vi "Dichtheitstest durchfuehren.vi"(8 "max. Druckanstieg":sgl, 9 "Wartezeit":sgl, 10 "Aktionen":T1=enum."Unterdruck aufbauen", 11 "Druck FT-IR":sgl) -> (0 "Status":string, 1 "Druckabfall":sgl, 2 "Aktionen":T1=enum."Unterdruck aufbauen", 3 "Verstrichene Zeit":sgl, 4 "Fehler":bool)   [LabVIEW 2020, in "Erweiterte Konfig.lvlib"]
uses:
  Erweiterte Konfig.lvlib
  Aktionen Dichtheitstest.ctl
  Schedule Modul/Aktion FGV Testdaten sammeln.ctl
  FGV PID Aktionen.ctl
  Sprachverwaltung/FGV Aktion Tabelle zerlegen.ctl
  Status Dichtheitstest Aktionen.ctl
  PNS/Aktionen FGV Grenzwerte.ctl
  Stoerungen/Stoerungen Messgeraet/Aktionen Kommunikation Stoerung.ctl
  FT-IR/FT-IR.lvlib
  Stoerungen/Stoerungen.lvlib
  Sprachverwaltung/Sprachverwaltung.lvlib
  Amium PNS/AK Kommunikation/AK Kommunikation.lvlib
  Amium PNS/AK Kommunikation/Amium Kommandos verwalten Aktionen.ctl
  Allgemein/allgemeine Sub-VIs.lvlib
  Schedule Modul/Schedule Modul.lvlib
  PNS/PNS.lvlib
  EPA 1065/Dichtheitstest 1065-345/Dichtheitstest 1065-345.lvlib
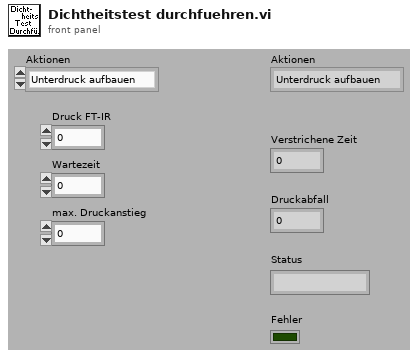
[diagram p1: front panel]
types:
  T1 = typedef "Erweiterte Konfig.lvlib/Aktionen Dichtheitstest.ctl" = enum16{"Initialisieren", "Unterdruck aufbauen", "Prop schließen", "Warten", "Auswertung", "Fertig"}
  T2 = typedef "PNS.lvlib/Aktionen FGV Grenzwerte.ctl" = enum16{"lesen", "Grenzw. schreiben", "Anweisungscode", "IP-Adresse", "laden", "speichern", "Anweisungscode vorgeben"}
  T3 = typedef "Erweiterte Konfig.lvlib/Status Dichtheitstest Aktionen.ctl" = enum16{"lesen", "Zeitstempel", "Daten", "läuft", "Protokolldaten"}
  T4 = typedef "Sprachverwaltung.lvlib/FGV Aktion Tabelle zerlegen.ctl" = enum16{"laden", "vereinzeln", "speichern"}
  T5 = typedef "Erweiterte Konfig.lvlib/FGV PID Aktionen.ctl" = enum16{"Lesen", "Schreiben PID", "Schreiben Sonstige", "Dichtheitstest", "Aktionen Dicht.", "Parameter Sensor"}
  T6 = typedef "Amium PNS.lvlib/AK Kommunikation.lvlib/Amium Kommandos verwalten Aktionen.ctl" = enum16{"lesen", "setzen Ende", "setzen Pos1", "senden", "initalisieren", "prüfen", "Kommandos"}
  T7 = typedef "Schedule Modul.lvlib/Aktion FGV Testdaten sammeln.ctl" = enum16{"lesen", "Dichtheitstest", "CalGasTest", "T90", "Kalibrieren", "init", "Kalender Daten"}
  T8 = typedef "Stoerungen.lvlib/Aktionen Kommunikation Stoerung.ctl" = enum16{"lesen", "init", "FT-IR Komm", "FT-IR Betriebsart", "FT-IR Hintergrund", "cRIO Komm", "PNS Komm", "Dichtheitstest", "Life Bit", "FTIR Komm AK", "PMA Komm", "FID Komm", "PMA Cal", "FID Ch4 Cal", "FID THC Cal", "Cal Timeout", "VFS 1 Komm", "VFS 2 Komm", "VFS 3 Komm", "VFS 4 Komm", "TRE 08 Komm", "CG-Test vorzeitig", "CG-Test Span 1", "CG-Test Span 2", "CG-Test Span 3", "CG-Test Messgas", "CG-Test löschen", "Test", "Amium AK", "AK Recept konfig", "AK Name konfig", "AK EKFG konfig"}
  T9 = typedef "Erweiterte Konfig.lvlib/Sonstige Parameter.ctl" = cluster{"Lüfter langsam":sgl, "Lüfter schnell":sgl, "FT-IR Kühlung Soll":sgl, "FT-IR Kühlung Max":sgl, "Überwachung":T10, "Befüllung aktiv":T11, "Stickstoff Befüllzeit":sgl, "Befüllintervall":sgl, "Kalibrierwert FT-IR":sgl, "Offset Ausgang":sgl, "Offset FT-IR":sgl, "Offset Druck FT-IR":sgl, "Dichtheitstest Zeit":sgl, "Dichtheitstest Abfall":sgl, "Dichtheitstest Umfang":T12, "Offset Umgebung":sgl, "Max Taupunkt":sgl, "Pumpendrehzahl":sgl, "ext. Befüllung":T11, "Ext. Stickstoff Befüllzeit":sgl}
  T10 = typedef "Auswahlfeld.ctl" = u16
  T11 = typedef "LogKonfig.lvlib/Auswahlfeld aktiviert-deaktiviert.ctl" = u16
  T12 = typedef "Erweiterte Konfig.lvlib/Dichtheitstest Umfang.ctl" = u16
  T13 = typedef "Erweiterte Konfig.lvlib/Dichtheitstest Protokoll.ctl" = cluster{"Startzeit":timestamp, "Endzeit":timestamp, "Startdruck":sgl, "Enddruck":sgl, "Dichtheitstest Umfang":T12}
  T14 = typedef "Schedule Modul.lvlib/Ergebnis Dichtheitstest.ctl" = cluster{"Druck FT-IR:":T15, "max. Anstieg:":T15, "Druckanstieg:":T15, "Zeitdauer:":T15, "Verstrichene Zeit:":T15, "Fehler":bool, "Unterdruck nicht erreicht ":bool}
  T15 = typedef "Zahlen-Ausgabefeld.ctl" = sgl
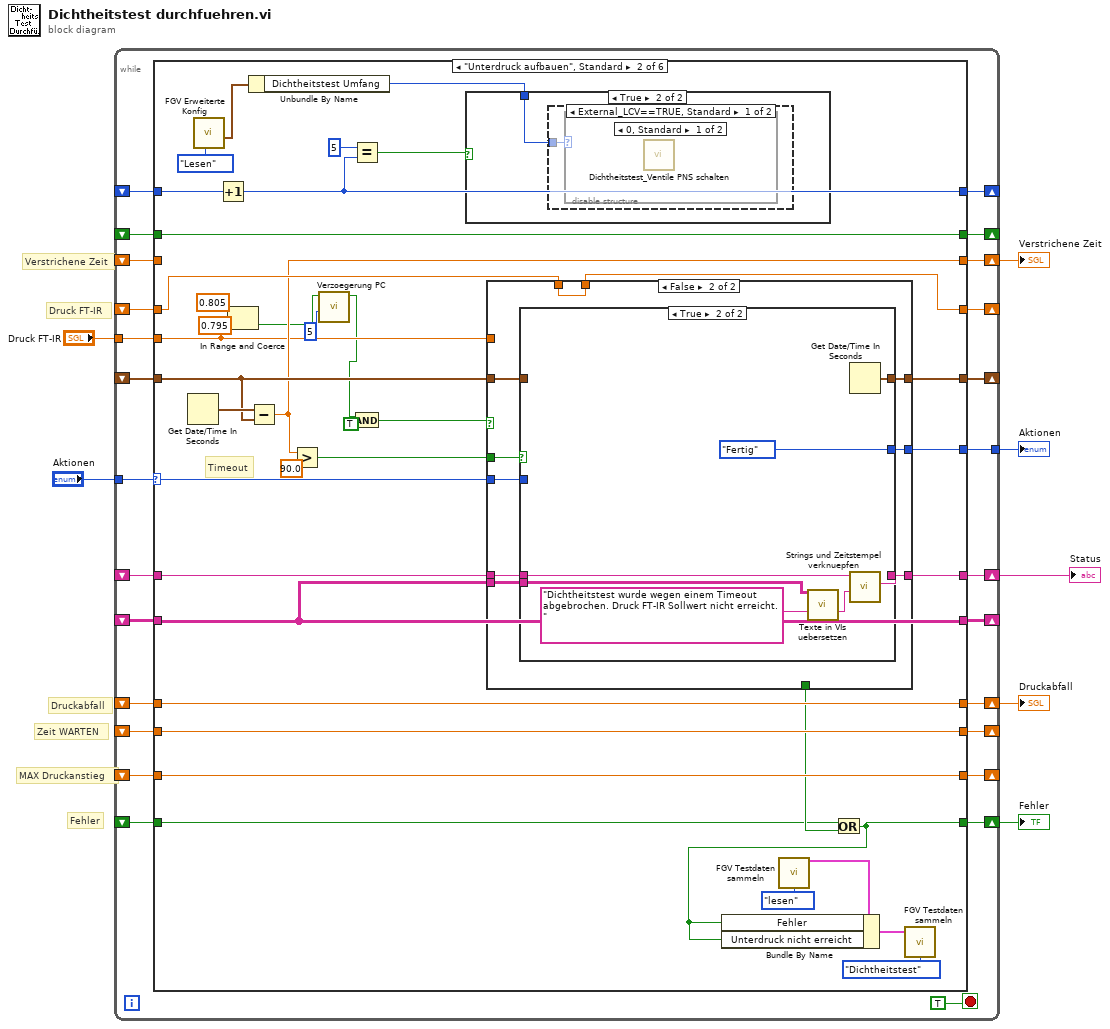
[diagram p0: block diagram]
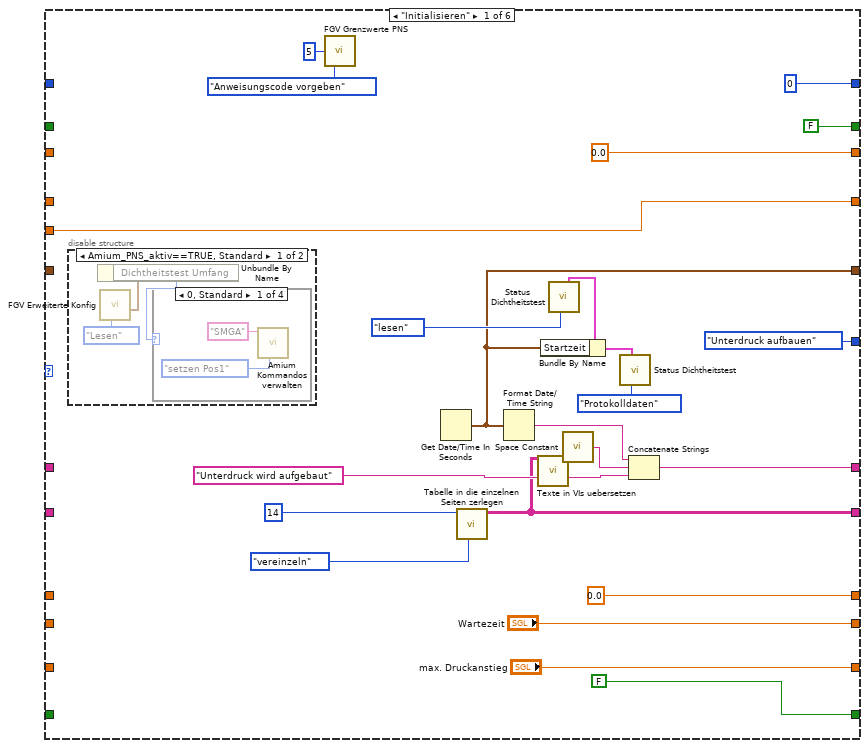
[diagram p2: hidden frame]
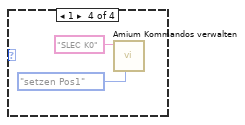
[diagram p5: hidden frame]
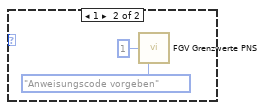
[diagram p8: hidden frame]
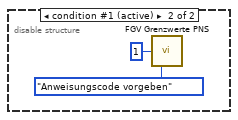
[diagram p9: hidden frame]
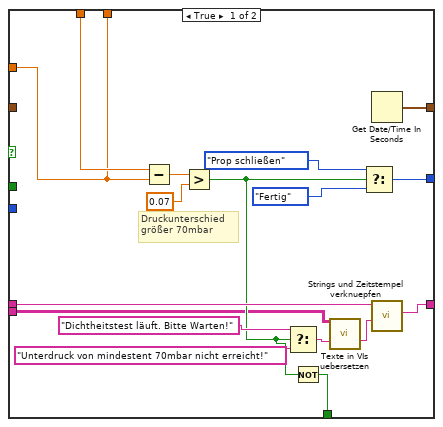
[diagram p10: hidden frame]
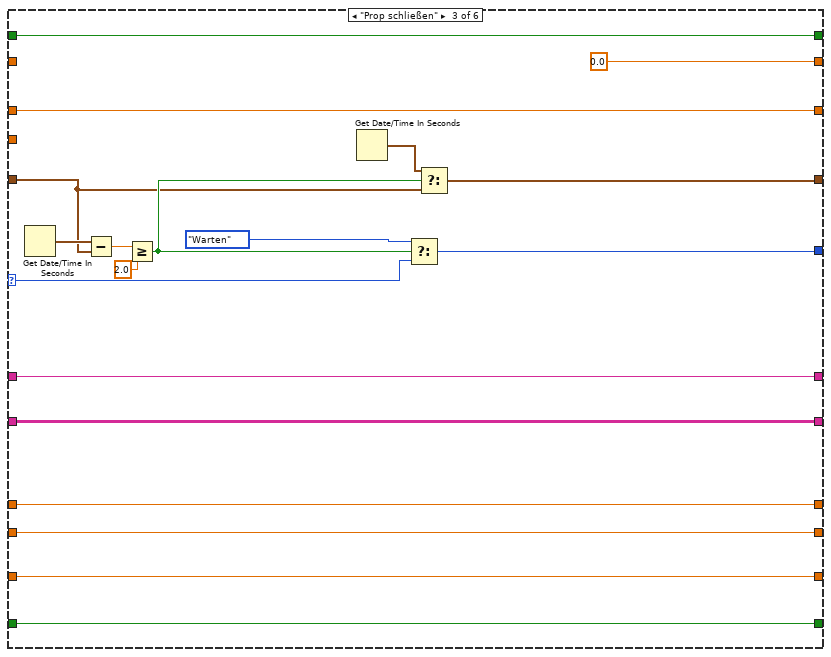
[diagram p12: hidden frame]
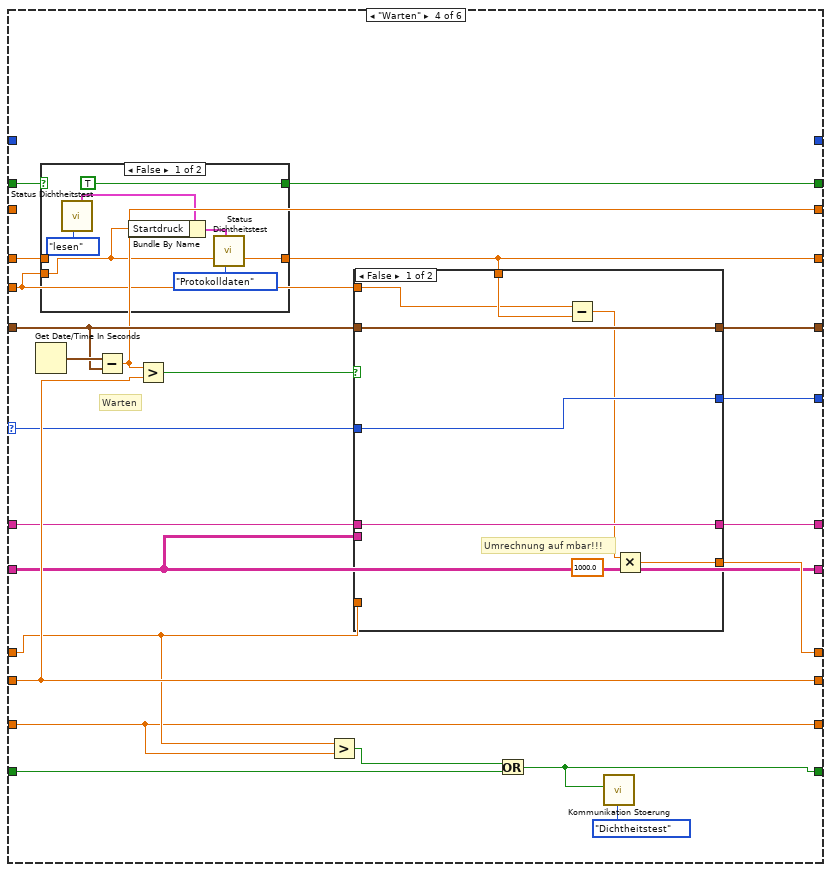
[diagram p13: hidden frame]
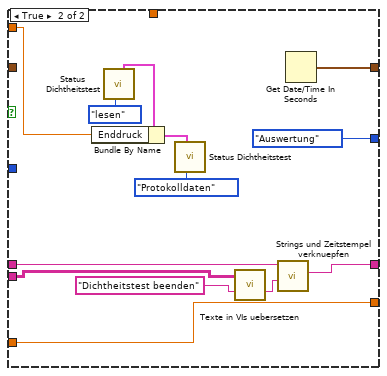
[diagram p15: hidden frame]
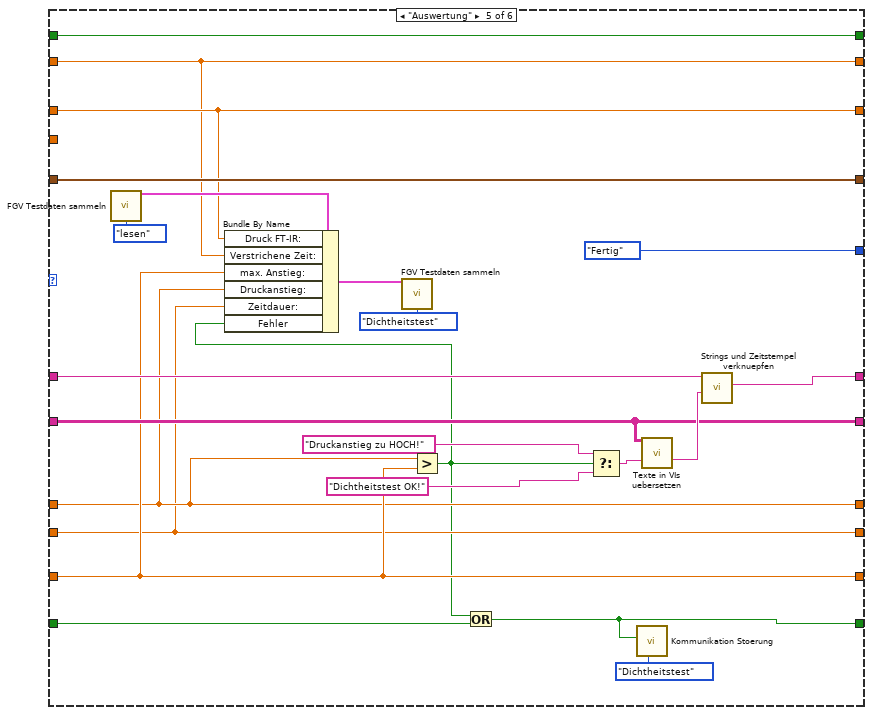
[diagram p16: hidden frame]
diagram:
  # "Verstrichene Zeit"
  # "Fehler"
  # "MAX Druckanstieg"
  # "Druckabfall"
  # "Zeit WARTEN"
  # "Druck FT-IR"
  n1 = while {
    shift-right: [w31] -> w1
    shift-left: _ -> [w30]
    tunnel: "Aktionen" -> [w32]
    tunnel: [w29] -> w6
    shift-right: [w28] -> _
    shift-left: _ -> [w27]
    shift-right: [w26] -> _
    shift-left: _ -> [w25]
    shift-right: [w23] -> _
    shift-left: _ -> [w21]
    shift-right: [w24] -> w5
    shift-left: _ -> [w22]
    shift-right: [w20] -> _
    shift-left: _ -> [w19]
    shift-right: [w18] -> w4
    shift-left: _ -> [w17]
    shift-right: [w15] -> w3
    shift-left: _ -> [w16]
    tunnel: "Druck FT-IR" -> [w14]
    shift-right: [w13] -> _
    shift-left: _ -> [w12]
    shift-right: [w11] -> _
    shift-left: _ -> [w10]
    shift-right: [w9] -> _
    shift-left: _ -> [w8]
    stop <- TRUE stop-if-true
    n2 = case shown="\"Unterdruck aufbauen\", Standard" w32 {
      selector: w32 -> [_ w94 w158 w182 _ w245]
      tunnel: [w48 w95 w156 w178 w237 w244] -> w31
      tunnel: w30 -> [_ w96 w156 w180 w236 w244]
      tunnel: [Aktionen_Dichtheitstest."Unterdruck aufbauen" ("Aktionen") w97 w157 w181 Aktionen_Dichtheitstest."Fertig" ("Aktionen") w245] -> w29
      tunnel: [w38 w100 w148 w183 w235 w246] -> w28
      tunnel: w27 -> [_ w101 w150 w184 w235 w246]
      tunnel: [w49 w98 w160 w166 w222 w247] -> w26
      tunnel: w25 -> [_ w99 w160 w167 w222 w247]
      tunnel: [sgl 0.0 w93 w155 w179 w219 w250] -> w24
      tunnel: ["Wartezeit" w92 w154 w186 w218 w249] -> w23
      tunnel: w22 -> [_ w93 w155 w176 w219 w250]
      tunnel: w21 -> [_ w92 w154 w186 w218 w249]
      tunnel: ["max. Druckanstieg" w91 w153 w175 w220 w248] -> w20
      tunnel: w19 -> [_ w91 w153 w175 w220 w248]
      tunnel: [sgl 0.0 w90 0.0 w177 w221 w243] -> w18
      tunnel: w17 -> [_ _ _ _ w221 w243]
      tunnel: w16 -> [_ w73 w152 w173 w233 w242]
      tunnel: [FALSE w72 w152 w171 w231 w242] -> w15
      tunnel: w14 -> [w49 w87 _ w165 _ _]
      tunnel: [w44 w89 w147 w170 w228 w241] -> w13
      tunnel: w12 -> [_ w89 w147 w170 w228 w241]
      tunnel: [FALSE w80 w146 w168 w227 w240] -> w11
      tunnel: w10 -> [_ w80 w146 w169 w227 w240]
      tunnel: [0 w70 _ _ _ _] -> w9
      tunnel: w8 -> [_ w71 _ _ _ _]
      frame "Initialisieren" {
        n3 = disable-structure shown="Amium_PNS_aktiv==TRUE, Standard" {
          frame condition #0 {
            n4 = call "FGV Erweiterte Konfig.vi"("Aktion"=FGV_PID_Aktionen."Lesen") -> ("Sonstige"=w59:T9)  [unwired: 5 in, 5 out]
            n5 = Unbundle By Name(w59) -> ("Dichtheitstest Umfang"=w58:T12)
            n6 = case shown="0, Standard" w58 {
              frame 0, Default {
                n7 = call "Amium Kommandos verwalten.vi"("Aktionen"=Amium_Kommandos_verwalten_Aktionen."setzen Pos1", "neues Kommando"="SMGA") -> ()  [unwired: 7 in, 3 out]
              }
              frame 3 {
              }
              frame 2 {
              }
              frame 1 {
                n8 = call "Amium Kommandos verwalten.vi"("Aktionen"=Amium_Kommandos_verwalten_Aktionen."setzen Pos1", "neues Kommando"="SLEC K0") -> ()  [unwired: 7 in, 3 out]
              }
            }
          }
          frame condition #1 (active) {
          }
        }
        n9 = call "FGV Grenzwerte PNS.vi"("Anweisungscode"=u16 5, "Aktionen FGV Grenzwerte"=Aktionen_FGV_Grenzwerte."Anweisungscode vorgeben") -> ()  [unwired: 11 in, 3 out]
        n10 = Get Date/Time In Seconds() -> (seconds since 1Jan1904=w38:timestamp)
        n11 = call "Tabelle in die einzelnen Seiten zerlegen.vi"("Aktion"=FGV_Aktion_Tabelle_zerlegen."vereinzeln", "Index (Seite)"=14) -> ("Sprachliste"=w44:string[][])  [unwired: 7 in, 2 out]
        n12 = Format Date/Time String(seconds (now)=w38) -> (date/time string=w56:string)  [unwired: 2 in]
        n13 = call "Texte in VIs uebersetzen.vi"("Sprachliste"=w44, "String zum Übersetzen"="Unterdruck wird aufgebaut" ("String")) -> ("String zum Übersetzen"=w46:string)  [unwired: 9 in, 4 out]
        n14 = call "Status Dichtheitstest.vi"("Aktionen"=Status_Dichtheitstest_Aktionen."lesen") -> ("Protokoll"=w41:T13)  [unwired: 6 in, 4 out]
        n15 = Bundle By Name(cluster=w41, "Startzeit"=w38) -> (w42:T13)
        n16 = call <vilib>:"Space Constant.vi"() -> ("String"=w57:string)
        n17 = call "Status Dichtheitstest.vi"("Aktionen"=Status_Dichtheitstest_Aktionen."Protokolldaten", "Protokoll"=w42) -> ()  [unwired: 5 in, 5 out]
        n18 = Concatenate Strings(w56, w57, w46) -> (w48:string)
      }
      frame "Unterdruck aufbauen", Default {
        # "Timeout"
        n19 = Get Date/Time In Seconds() -> (seconds since 1Jan1904=w103:timestamp)
        n20 = call "FGV Erweiterte Konfig.vi"("Aktion"=FGV_PID_Aktionen."Lesen") -> ("Sonstige"=w66:T9)  [unwired: 5 in, 5 out]
        n21 = Increment(x=w71) -> (x+1=w70:i32)
        n22 = In Range and Coerce(upper limit=0.805 ("Obergrenze"), x=w87, lower limit=0.795 ("Obergrenze")) -> (In Range?=w84:bool)  [unwired: 1 out]
        n23 = Unbundle By Name(w66) -> ("Dichtheitstest Umfang"=w65:T12)
        n24 = Subtract(x=w103, y=w101) -> (x-y=w90:dbl)
        n25 = Greater?(x=w90, y=90.0) -> (0:w79:bool)
        n26 = call "Verzoegerung PC.vi"("sec"=u16 5, "Startsignal"=w84) -> ("Zeit abgelaufen?"=w83:bool)  [unwired: 8 in, 1 out]
        n27 = Equal?(x=5, y=w70) -> (x = y?=w68:bool)
        n28 = And(x=w83, y=TRUE) -> (x .and. y?=w85:bool)
        n29 = case shown="True" w68 {
          tunnel: w65 -> [_ w104]
          frame False {
          }
          frame True {
            n30 = disable-structure shown="External_LCV==TRUE, Standard" {
              disable-tunnel: w104 -> [w105 _]
              frame condition #0 {
                n31 = case shown="0, Standard" w105 {
                  frame 0, Default {
                    n32 = call "Dichtheitstest_Ventile PNS schalten.vi"() -> ()  [unwired: 11 in, 1 out]
                  }
                  frame 1 {
                    n33 = call "FGV Grenzwerte PNS.vi"("Anweisungscode"=u16 1, "Aktionen FGV Grenzwerte"=Aktionen_FGV_Grenzwerte."Anweisungscode vorgeben") -> ()  [unwired: 11 in, 3 out]
                  }
                }
              }
              frame condition #1 (active) {
                n34 = call "FGV Grenzwerte PNS.vi"("Anweisungscode"=u16 1, "Aktionen FGV Grenzwerte"=Aktionen_FGV_Grenzwerte."Anweisungscode vorgeben") -> ()  [unwired: 11 in, 3 out]
              }
            }
          }
        }
        n35 = case shown="False" w85 {
          tunnel: w101 -> [_ w128]
          tunnel: [w126 w135] -> w100
          tunnel: w99 -> [w125 w129]
          tunnel: [w110 w129] -> w98
          tunnel: [w120 w134] -> w97
          tunnel: w96 -> [w119 w133]
          tunnel: [w118 w132] -> w95
          tunnel: w94 -> [_ w127]
          tunnel: [w114 _] -> w74
          tunnel: w87 -> [w110 _]
          tunnel: w89 -> [w111 w131]
          tunnel: w79 -> [_ w130]
          frame True {
            # "Druckunterschied \ngrößer 70mbar"
            n36 = Subtract(x=w125, y=w110) -> (x-y=w124:sgl)
            n37 = Greater?(x=w124, y=0.07) -> (0:w115:bool)
            n38 = Select(t="Dichtheitstest läuft. Bitte Warten!" ("String"), s=w115, f="Unterdruck von mindestent 70mbar nicht erreicht!" ("String")) -> (s? t:f=w113:string)
            n39 = Not(x=w115) -> (.not. x?=w114:bool)
            n40 = call "Texte in VIs uebersetzen.vi"("Sprachliste"=w111, "String zum Übersetzen"=w113) -> ("String zum Übersetzen"=w112:string)  [unwired: 9 in, 4 out]
            n41 = Select(t=Aktionen_Dichtheitstest."Prop schließen" ("Aktionen"), s=w115, f=Aktionen_Dichtheitstest."Fertig" ("Aktionen")) -> (s? t:f=w120:T1)
            n42 = Get Date/Time In Seconds() -> (seconds since 1Jan1904=w126:timestamp)
            n43 = call "Strings und Zeitstempel verknuepfen.vi"("String 1 hinzufügen"=w112, "Eingagns String"=w119) -> ("Verknüpfter String"=w118:string)  [unwired: 9 in]
          }
          frame False {
            n44 = case shown="True" w130 {
              tunnel: [w137 w145] -> w135
              tunnel: [w136 Aktionen_Dichtheitstest."Fertig" ("Aktionen")] -> w134
              tunnel: w133 -> [w138 w143]
              tunnel: [w138 w142] -> w132
              tunnel: w131 -> [_ w140]
              tunnel: w128 -> [w137 _]
              tunnel: w127 -> [w136 _]
              frame False {
              }
              frame True {
                n45 = call "Texte in VIs uebersetzen.vi"("Sprachliste"=w140, "String zum Übersetzen"="Dichtheitstest wurde wegen einem Timeout abgebrochen. Druck FT-IR Sollwert nicht erreicht." ("String")) -> ("String zum Übersetzen"=w141:string)  [unwired: 9 in, 4 out]
                n46 = Get Date/Time In Seconds() -> (seconds since 1Jan1904=w145:timestamp)
                n47 = call "Strings und Zeitstempel verknuepfen.vi"("String 1 hinzufügen"=w141, "Eingagns String"=w143) -> ("Verknüpfter String"=w142:string)  [unwired: 9 in]
              }
            }
          }
        }
        n48 = call "FGV Testdaten sammeln.vi"("Aktion"=Aktion_FGV_Testdaten_sammeln."lesen") -> ("Ergebnisse Dichtheitstest"=w77:T14)  [unwired: 9 in, 5 out]
        n49 = Or(x=w73, y=w74) -> (x .or. y?=w72:bool)
        n50 = Bundle By Name(cluster=w77, "Fehler"=w72, "Unterdruck nicht erreicht"=w72) -> (w75:T14)
        n51 = call "FGV Testdaten sammeln.vi"("Ergebnisse Dichtheitstest"=w75, "Aktion"=Aktion_FGV_Testdaten_sammeln."Dichtheitstest") -> ()  [unwired: 8 in, 6 out]
      }
      frame "Prop schließen" {
        n52 = Get Date/Time In Seconds() -> (seconds since 1Jan1904=w164:timestamp)
        n53 = Subtract(x=w164, y=w150) -> (x-y=w163:dbl)
        n54 = Greater Or Equal?(x=w163, y=2.0) -> (x >= y?=w151:bool)
        n55 = Get Date/Time In Seconds() -> (seconds since 1Jan1904=w149:timestamp)
        n56 = Select(t=Aktionen_Dichtheitstest."Warten" ("Aktionen"), s=w151, f=w158) -> (s? t:f=w157:T1)
        n57 = Select(t=w149, s=w151, f=w150) -> (s? t:f=w148:timestamp)
      }
      frame "Warten" {
        # "Warten"
        n58 = Get Date/Time In Seconds() -> (seconds since 1Jan1904=w187:timestamp)
        n59 = case shown="False" w169 {
          selector: w169 -> [_ w195]
          tunnel: [TRUE w195] -> w168
          tunnel: w167 -> [_ w194]
          tunnel: [w188 w194] -> w166
          tunnel: w165 -> [w188 _]
          frame False {
            n60 = call "Status Dichtheitstest.vi"("Aktionen"=Status_Dichtheitstest_Aktionen."lesen") -> ("Protokoll"=w189:T13)  [unwired: 6 in, 4 out]
            n61 = Bundle By Name(cluster=w189, "Startdruck"=w188) -> (w192:T13)
            n62 = call "Status Dichtheitstest.vi"("Aktionen"=Status_Dichtheitstest_Aktionen."Protokolldaten", "Protokoll"=w192) -> ()  [unwired: 5 in, 5 out]
          }
          frame True {
          }
        }
        n63 = Subtract(x=w187, y=w184) -> (x-y=w177:dbl)
        n64 = Greater?(x=w177, y=w186) -> (0:w185:bool)
        n65 = Greater?(x=w176, y=w175) -> (0:w174:bool)
        n66 = case shown="False" w185 {
          tunnel: w184 -> [w203 _]
          tunnel: [w203 w215] -> w183
          tunnel: w182 -> [w202 _]
          tunnel: [w202 Aktionen_Dichtheitstest."Auswertung" ("Aktionen")] -> w181
          tunnel: w180 -> [w201 w214]
          tunnel: w176 -> [_ w213]
          tunnel: [w199 w213] -> w179
          tunnel: [w201 w212] -> w178
          tunnel: w166 -> [w197 _]
          tunnel: w165 -> [w196 w204]
          tunnel: w170 -> [_ w209]
          frame False {
            # "Umrechnung auf mbar!!!"
            n67 = Subtract(x=w196, y=w197) -> (x-y=w198:sgl)
            n68 = Multiply(x=w198, y=sgl 1000.0) -> (x*y=w199:sgl)
          }
          frame True {
            n69 = call "Status Dichtheitstest.vi"("Aktionen"=Status_Dichtheitstest_Aktionen."lesen") -> ("Protokoll"=w207:T13)  [unwired: 6 in, 4 out]
            n70 = Bundle By Name(cluster=w207, "Enddruck"=w204) -> (w208:T13)
            n71 = call "Status Dichtheitstest.vi"("Aktionen"=Status_Dichtheitstest_Aktionen."Protokolldaten", "Protokoll"=w208) -> ()  [unwired: 5 in, 5 out]
            n72 = call "Texte in VIs uebersetzen.vi"("Sprachliste"=w209, "String zum Übersetzen"="Dichtheitstest beenden" ("String")) -> ("String zum Übersetzen"=w210:string)  [unwired: 9 in, 4 out]
            n73 = call "Strings und Zeitstempel verknuepfen.vi"("String 1 hinzufügen"=w210, "Eingagns String"=w214) -> ("Verknüpfter String"=w212:string)  [unwired: 9 in]
            n74 = Get Date/Time In Seconds() -> (seconds since 1Jan1904=w215:timestamp)
          }
        }
        n75 = Or(x=w174, y=w173) -> (x .or. y?=w171:bool)
        n76 = call "Kommunikation Stoerung.vi"("Aktionen"=Aktionen_Kommunikation_Stoerung."Dichtheitstest", "ERROR"=w171) -> ()  [unwired: 9 in, 1 out]
      }
      frame "Auswertung" {
        n77 = call "FGV Testdaten sammeln.vi"("Aktion"=Aktion_FGV_Testdaten_sammeln."lesen") -> ("Ergebnisse Dichtheitstest"=w224:T14)  [unwired: 9 in, 5 out]
        n78 = Greater?(x=w219, y=w220) -> (0:w217:bool)
        n79 = Bundle By Name(cluster=w224, "Druck FT-IR:"=w222, "Verstrichene Zeit:"=w221, "max. Anstieg:"=w220, "Druckanstieg:"=w219, "Zeitdauer:"=w218, "Fehler"=w217) -> (w223:T14)
        n80 = call "FGV Testdaten sammeln.vi"("Ergebnisse Dichtheitstest"=w223, "Aktion"=Aktion_FGV_Testdaten_sammeln."Dichtheitstest") -> ()  [unwired: 8 in, 6 out]
        n81 = Or(x=w217, y=w233) -> (x .or. y?=w231:bool)
        n82 = Select(t="Druckanstieg zu HOCH!" ("String"), s=w217, f="Dichtheitstest OK!" ("String")) -> (s? t:f=w230:string)
        n83 = call "Kommunikation Stoerung.vi"("Aktionen"=Aktionen_Kommunikation_Stoerung."Dichtheitstest", "ERROR"=w231) -> ()  [unwired: 9 in, 1 out]
        n84 = call "Texte in VIs uebersetzen.vi"("Sprachliste"=w228, "String zum Übersetzen"=w230) -> ("String zum Übersetzen"=w229:string)  [unwired: 9 in, 4 out]
        n85 = call "Strings und Zeitstempel verknuepfen.vi"("String 1 hinzufügen"=w229, "Eingagns String"=w236) -> ("Verknüpfter String"=w237:string)  [unwired: 9 in]
      }
      frame "Fertig" {
      }
    }
  }
  "Aktionen" <- w6
  "Status" <- w1
  "Druckabfall" <- w5
  "Verstrichene Zeit" <- w4
  "Fehler" <- w3
